vi "ConvertToTable.vi"(6 "Conf. Gral.":T1, 8 "error in (no error)":errorcluster, 9 "Array Parsed Expression In":T2[](array[typedef]), 10 "Dcte":sgl[](array[numeric]), 11 "Kcte":sgl[](array[numeric])) -> (0 "error out":errorcluster, 3 "Mediciones":string[][](array[string]))   [LabVIEW 2014, in "ConfigProg.lvlib"]
doc: "Convierte los datos de Ctes, Dimensiones y arma el Array Parsed Expression(1D array) en la tabla de Mediciones (2D array)."
uses:
  ConfigProg.lvlib
  TypeDefs/ParsedExpression.ctl
  TypeDefs/typeMed.ctl
  TypeDefs/Conf. Gral.ctl
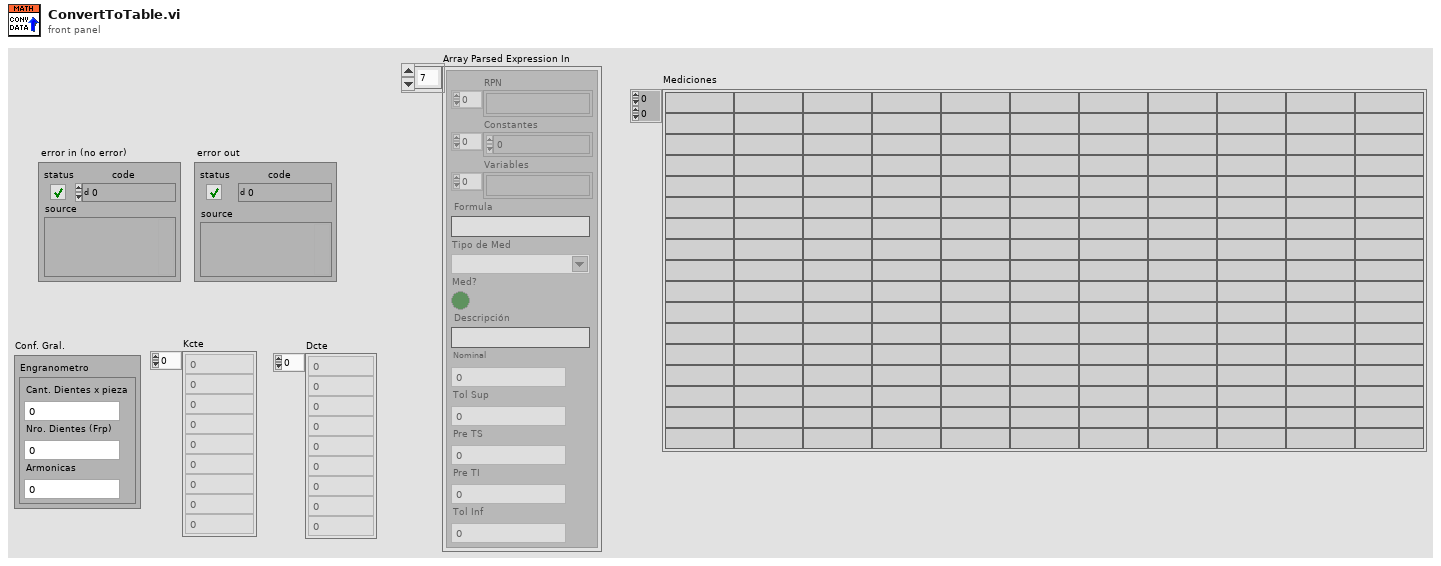
[diagram p1: front panel]
types:
  T1 = typedef "ConfigProg.lvlib/Conf. Gral.ctl" = cluster{"Engranometro":cluster{"Cant. Dientes x pieza":i32, "Nro. Dientes (Frp)":i32, "Armonicas":i32}}
  T2 = typedef "ConfigProg.lvlib/ParsedExpression.ctl" = cluster{"RPN ":string[], "Constantes":sgl[], "Variables":string[], "Formula":string, "Tipo de Med":T3, "Med?":bool, "Descripción":string, "Nominal":sgl, "Tol Sup":sgl, "Pre TS":sgl, "Pre TI":sgl, "Tol Inf":sgl}
  T3 = typedef "ConfigProg.lvlib/typeMed.ctl" = string
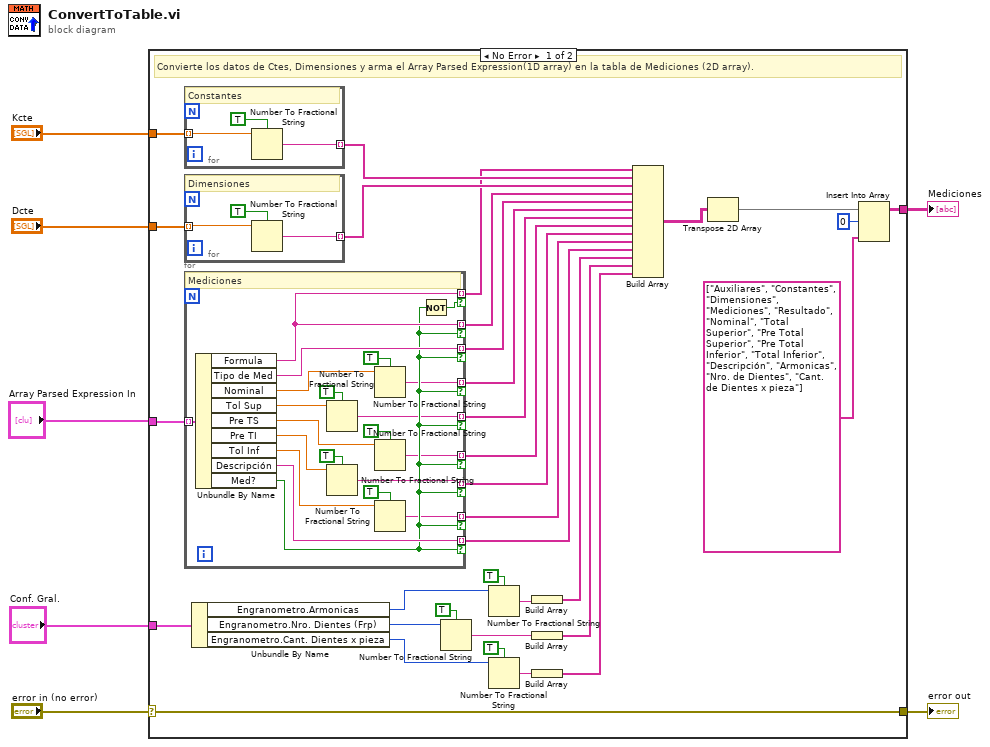
[diagram p0: block diagram]
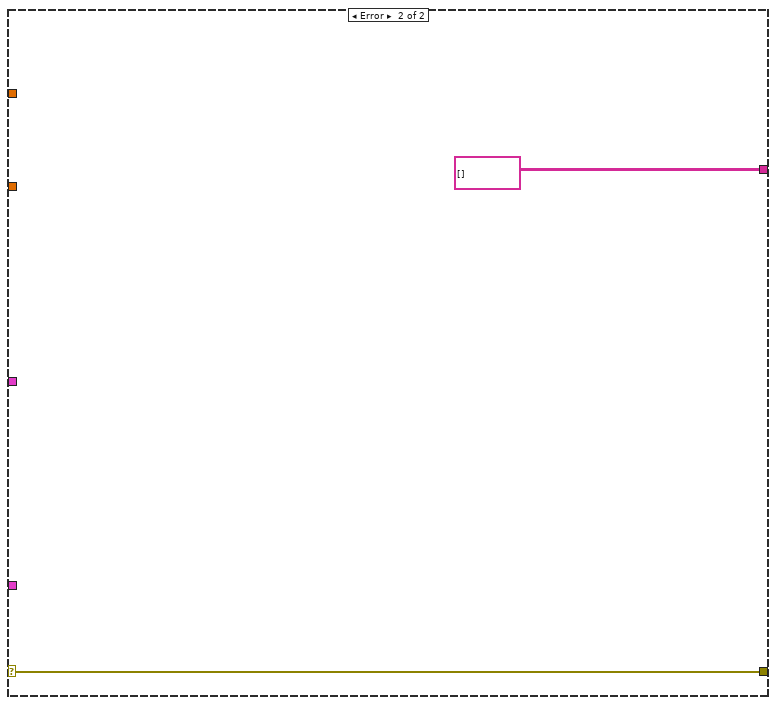
[diagram p2: hidden frame]
diagram:
  n1 = case shown="No Error" "error in (no error)" {
    selector: "error in (no error)" -> [w40 w69]
    tunnel: [w40 w69] -> w6
    tunnel: "Array Parsed Expression In" -> [w39 _]
    tunnel: "Kcte" -> [w38 _]
    tunnel: "Dcte" -> [w37 _]
    tunnel: [w23 T3[][] []] -> w2
    tunnel: "Conf. Gral." -> [w20 _]
    frame No Error {
      # "Convierte los datos de Ctes, Dimensiones y arma el Array Parsed Expression(1D array) en la tabla de Mediciones (2D array)."
      n2 = for {
        tunnel: w38 -> [w43] mode=indexing
        tunnel: [w41] -> w36 mode=indexing
        # "Constantes"
        n3 = Number To Fractional String(use system decimal point (T)=TRUE, number=w43) -> (F-format string=w41:string)  [unwired: 2 in]
      }
      n4 = for {
        tunnel: w37 -> [w45] mode=indexing
        tunnel: [w44] -> w35 mode=indexing
        # "Dimensiones"
        n5 = Number To Fractional String(use system decimal point (T)=TRUE, number=w45) -> (F-format string=w44:string)  [unwired: 2 in]
      }
      n6 = for {
        tunnel: [w66] -> w31 mode=indexing if=w62
        tunnel: w39 -> [w67] mode=indexing
        tunnel: [w56] -> w26 mode=indexing if=w62
        tunnel: [w54] -> w27 mode=indexing if=w62
        tunnel: [w53] -> w28 mode=indexing if=w62
        tunnel: [w52] -> w29 mode=indexing if=w62
        tunnel: [w51] -> w30 mode=indexing if=w62
        tunnel: [w65] -> w32 mode=indexing if=w62
        tunnel: [w64] -> w33 mode=indexing if=w62
        tunnel: [w64] -> w34 mode=indexing if=w63
        # "Mediciones"
        n7 = Unbundle By Name(w67) -> ("Formula"=w64:string, "Tipo de Med"=w65:T3, "Nominal"=w50:sgl, "Tol Sup"=w49:sgl, "Pre TS"=w48:sgl, "Pre TI"=w47:sgl, "Tol Inf"=w55:sgl, "Descripción"=w66:string, "Med?"=w62:bool)
        n8 = Number To Fractional String(use system decimal point (T)=TRUE, number=w49) -> (F-format string=w52:string)  [unwired: 2 in]
        n9 = Number To Fractional String(use system decimal point (T)=TRUE, number=w47) -> (F-format string=w54:string)  [unwired: 2 in]
        n10 = Number To Fractional String(use system decimal point (T)=TRUE, number=w50) -> (F-format string=w51:string)  [unwired: 2 in]
        n11 = Number To Fractional String(use system decimal point (T)=TRUE, number=w48) -> (F-format string=w53:string)  [unwired: 2 in]
        n12 = Number To Fractional String(use system decimal point (T)=TRUE, number=w55) -> (F-format string=w56:string)  [unwired: 2 in]
        n13 = Not(x=w62) -> (.not. x?=w63:bool)
      }
      n14 = Unbundle By Name(w20) -> ("Engranometro.Armonicas"=w16:i32, "Engranometro.Nro. Dientes (Frp)"=w15:i32, "Engranometro.Cant. Dientes x pieza"=w14:i32)
      n15 = Number To Fractional String(use system decimal point (T)=TRUE, number=w15) -> (F-format string=w11:string)  [unwired: 2 in]
      n16 = Number To Fractional String(use system decimal point (T)=TRUE, number=w16) -> (F-format string=w12:string)  [unwired: 2 in]
      n17 = Number To Fractional String(use system decimal point (T)=TRUE, number=w14) -> (F-format string=w9:string)  [unwired: 2 in]
      n18 = Build Array(w12) -> (w13:string[])
      n19 = Build Array(w11) -> (w10:string[])
      n20 = Build Array(w9) -> (w8:string[])
      n21 = Build Array(w34, w36, w35, w33, w32, w30, w29, w28, w27, w26, w31, w13, w10, w8) -> (w25:T3[][])
      n22 = Transpose 2D Array(2D array=w25) -> (transposed array=w24:T3[][])
      n23 = Insert Into Array(array=w24, index (row)=0, new element=string[] ["Auxiliares", "Constantes", "Dimensiones", "Mediciones", "Resultado", "Nominal", "Total Superior", "Pre Total Superior", "Pre Total Inferior", "Total Inferior", "Descripción", "Armonicas", "Nro. de Dientes", "Cant. de Dientes x pieza"] ("new element/subarray")) -> (w23:T3[][])  [unwired: 1 in]
    }
    frame Error {
    }
  }
  "Mediciones" <- w2
  "error out" <- w6
